vi "蠕动泵组合启动命令.vi"(8 "Error in":errorcluster caption="Error in (no error)", 10 "控制方式":T1(ring)=enum."进样停止", 11 "仪器":enum16{"", "氨氮", "总磷", "总氮", "CODMn", "CODCr"}(ring)=enum."氨氮") -> (0 "error out":errorcluster)   [LabVIEW 2016, in "质控单元.lvlib"]
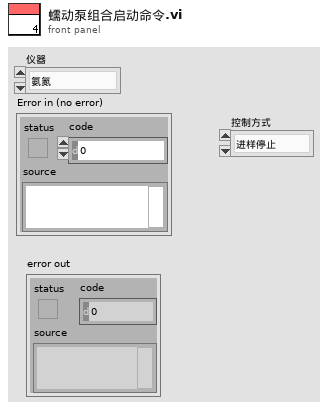
[diagram p1: front panel]
types:
  T1 = enum16{"进样", "进样停止", "排液", "排液停止", "搅拌", "搅拌停止", "定量", "定量停止"}
  T2 = enum16{"打开三通阀", "关闭三通阀", "蠕动泵正转", "蠕动泵反转", "蠕动泵停止", "进水样", "排废液", "进空气"}
  T3 = enum16{"打开三通阀", "关闭三通阀", "蠕动泵正转", "蠕动泵反转", "蠕动泵停止"}
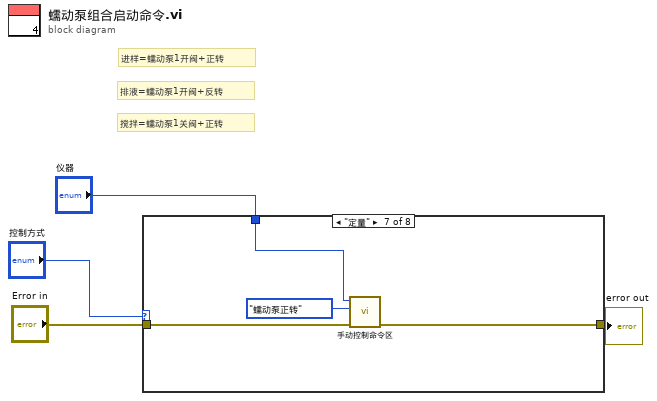
[diagram p0: block diagram]
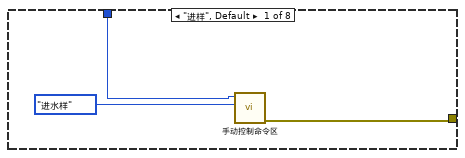
[diagram p2: hidden frame]
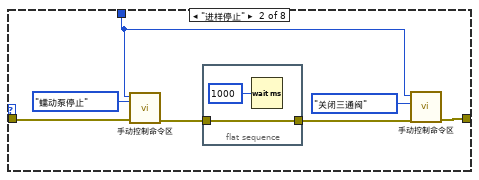
[diagram p3: hidden frame]
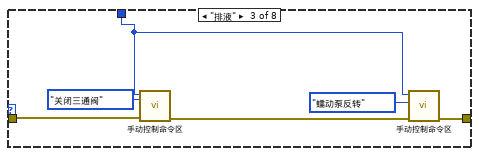
[diagram p4: hidden frame]
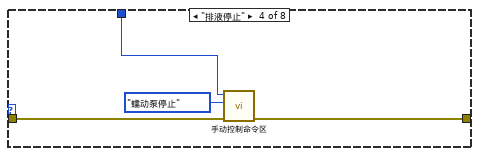
[diagram p5: hidden frame]
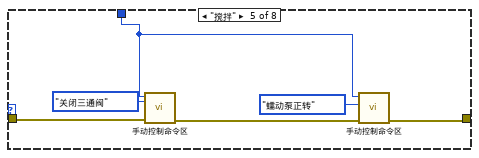
[diagram p6: hidden frame]
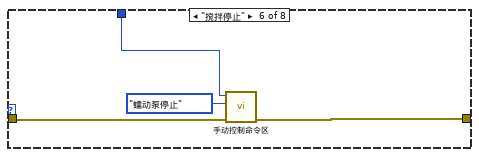
[diagram p7: hidden frame]
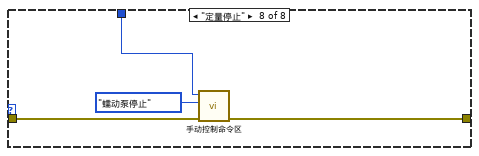
[diagram p8: hidden frame]
diagram:
  # "搅拌=蠕动泵1关阀+正转"
  # "排液=蠕动泵1开阀+反转"
  # "进样=蠕动泵1开阀+正转"
  n1 = case shown="\"定量\"" "控制方式" {
    tunnel: "仪器" -> [w6 w11 w18 w25 w28 w35 w40 w43]
    tunnel: "Error in" -> [_ w12 w19 w24 w29 w34 w39 w42]
    tunnel: [w5 w10 w17 w23 w27 w33 w38 w41] -> w2
    frame "进样", Default {
      n2 = call-poly "手动控制命令区.vi"("启动命令"=T2."进水样", "仪器"=w6) -> ("error out"=w5:errorcluster)  [unwired: 9 in]
    }
    frame "进样停止" {
      n3 = call-poly "手动控制命令区.vi"("Error in"=w12, "启动命令"=T2."蠕动泵停止", "仪器"=w11) -> ("error out"=w9:errorcluster)  [unwired: 8 in]
      n4 = flat-sequence {
        tunnel: w9 -> [w15]
        tunnel: [w15] -> w8
        frame #0 {
          n5 = Wait (ms)(milliseconds to wait=u32 1000 ("等待时间（毫秒）")) -> ()  [unwired: 1 out]
        }
      }
      n6 = call-poly "手动控制命令区.vi"("Error in"=w8, "启动命令"=T2."关闭三通阀", "仪器"=w11) -> ("error out"=w10:errorcluster)  [unwired: 8 in]
    }
    frame "排液" {
      n7 = call-poly "手动控制命令区.vi"("Error in"=w19, "启动命令"=T2."关闭三通阀", "仪器"=w18) -> ("error out"=w20:errorcluster)  [unwired: 8 in]
      n8 = call-poly "手动控制命令区.vi"("Error in"=w20, "启动命令"=T2."蠕动泵反转", "仪器"=w18) -> ("error out"=w17:errorcluster)  [unwired: 8 in]
    }
    frame "排液停止" {
      n9 = call-poly "手动控制命令区.vi"("Error in"=w24, "启动命令"=T2."蠕动泵停止", "仪器"=w25) -> ("error out"=w23:errorcluster)  [unwired: 8 in]
    }
    frame "搅拌" {
      n10 = call-poly "手动控制命令区.vi"("Error in"=w29, "启动命令"=T2."关闭三通阀", "仪器"=w28) -> ("error out"=w30:errorcluster)  [unwired: 8 in]
      n11 = call-poly "手动控制命令区.vi"("Error in"=w30, "启动命令"=T2."蠕动泵正转", "仪器"=w28) -> ("error out"=w27:errorcluster)  [unwired: 8 in]
    }
    frame "搅拌停止" {
      n12 = call-poly "手动控制命令区.vi"("Error in"=w34, "启动命令"=T2."蠕动泵停止", "仪器"=w35) -> ("error out"=w33:errorcluster)  [unwired: 8 in]
    }
    frame "定量" {
      n13 = call-poly "手动控制命令区.vi"("Error in"=w39, "启动命令"=T3."蠕动泵正转", "仪器"=w40) -> ("error out"=w38:errorcluster)  [unwired: 8 in]
    }
    frame "定量停止" {
      n14 = call-poly "手动控制命令区.vi"("Error in"=w42, "启动命令"=T3."蠕动泵停止", "仪器"=w43) -> ("error out"=w41:errorcluster)  [unwired: 8 in]
    }
  }
  "error out" <- w2
